vi "Write Graph.vi"(8 "error in (no error)":errorcluster, 10 "Graph":refnum<class "Graph.lvclass">, 11 "Topological Sort in":refnum<class "Topological Sort.lvclass">) -> (0 "error out":errorcluster, 3 "Topological Sort out":refnum<class "Topological Sort.lvclass">)   [LabVIEW 2025, in "AOC.lvlib" / "Topological Sort.lvlib" / "Topological Sort.lvclass"]
uses:
  Topological Sort.lvclass
  Graph/Graph.lvclass
  Topological Sort.lvclass/Topological Sort.ctl
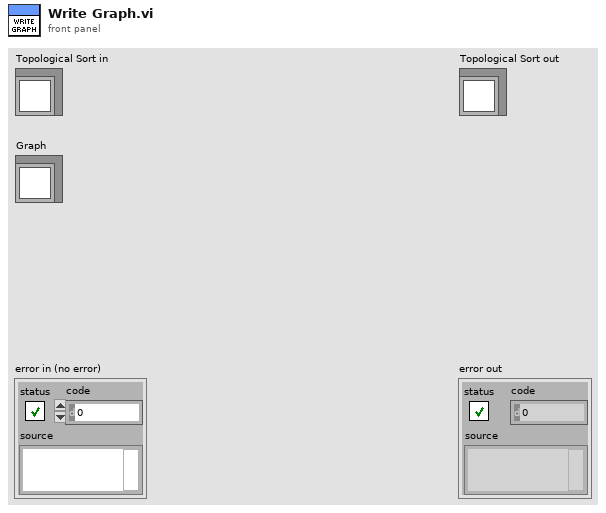
[diagram p1: front panel]
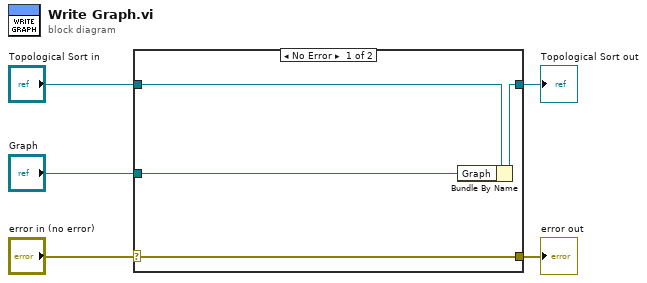
[diagram p0: block diagram]
diagram:
  n1 = case shown="No Error" "error in (no error)" {
    selector: "error in (no error)" -> [w9 w10]
    tunnel: [w9 w10] -> w4
    tunnel: [w7 w11] -> w2
    tunnel: "Topological Sort in" -> [w8 w11]
    tunnel: "Graph" -> [w6 _]
    frame No Error {
      n2 = Bundle By Name(cluster=w8, "Graph"=w6) -> (w7:refnum<class "Topological Sort.lvclass">)
    }
    frame Error {
    }
  }
  "error out" <- w4
  "Topological Sort out" <- w2
